vi "Acc G test.vi"() -> ()   [LabVIEW 2013]
uses:
  <vilib>/Utility/error.llb/DialogType.ctl
  <vilib>/DAQmx/read.llb/DAQmx Read (Analog 1D Wfm NChan NSamp).vi
  <vilib>/DAQmx/configure/timing.llb/DAQmx Timing (Sample Clock).vi
  <vilib>/DAQmx/configure/task.llb/DAQmx Configure Logging (TDMS).vi
  <vilib>/measure/mascope.llb/Transition Measurements N chan.vi
  <vilib>/DAQmx/create/channels.llb/DAQmx Create Channel (AI-Voltage-Basic).vi
  <vilib>/DAQmx/configure/trigger.llb/DAQmx Start Trigger (Digital Edge).vi
  <vilib>/DAQmx/configure/trigger.llb/DAQmx Start Trigger (Analog Edge).vi
  <vilib>/DAQmx/configure/trigger.llb/DAQmx Reference Trigger (Digital Edge).vi
  <vilib>/DAQmx/configure/trigger.llb/DAQmx Reference Trigger (Analog Edge).vi
  <vilib>/DAQmx/miscellaneous.llb/DAQmx Fill In Error Info.vi
  <resource>/objmgr/daqmx.rc
  <vilib>/measure/NI_MAPro.lvlib
panel:
  out "Y max":dbl caption="Y 최대" format="%0.2f"
  out "웨이브폼 그래프":waveform(dbl)[](graph)
  in  "샘플 개수":i32=100
  in  "트리거 타입":T1(tab)
  in  "에지":i32(ring)=10280 items=["상승"=10280, "하강"=10171]
  in  "디지털 트리거 소스":tag
  in  "레벨(V)":dbl format="%0.2f"
  in  "히스테리시스(V)":dbl
  in  "기울기":i32(ring)=10280 items=["상승"=10280, "하강"=10171]
  in  "아날로그 트리거 소스":string="APFI0"
  in  "디지털 참조 트리거 소스":tag
  in  "에지 2":i32(ring)=10280 items=["상승"=10280, "하강"=10171]
  in  "트리거 이전 샘플":u32
  in  "아날로그 참조 트리거 소스":string="APFI0"
  in  "기울기 2":i32(ring)=10280 items=["상승"=10280, "하강"=10171]
  in  "레벨(V) 2":dbl format="%0.2f"
  in  "트리거 이전 샘플 2":u32
  in  "TDMS 파일 경로":path
  in  "샘플 속도":dbl=1000.0
  in  "샘플 클럭 소스":tag="OnboardClock"
  in  "터미널 설정":i32(ring)=-1 items=["기본값"=-1, "RSE"=10083, "NRSE"=10078, "차동"=10106, "유사 차동"=12529]
  in  "최대 전압":dbl=5.0
  in  "최소 전압":dbl=-5.0
  in  "물리적인 채널":tag="Dev1/ai0"
  out "실제 샘플 속도":dbl=1000.0 format="%0.2f"
  in  "로깅 모드":i32(ring)=10231 items=["Off"=10231, "로그 및 읽기"=15842]
  # "시작 트리거를 설정하고 사용하려면 위의 탭이 있어야 합니다.  일부 하드웨어는 트리거를 지원하지 않습니다. 더 자세한 정보는 디바이스 문서를 참조하십시오."
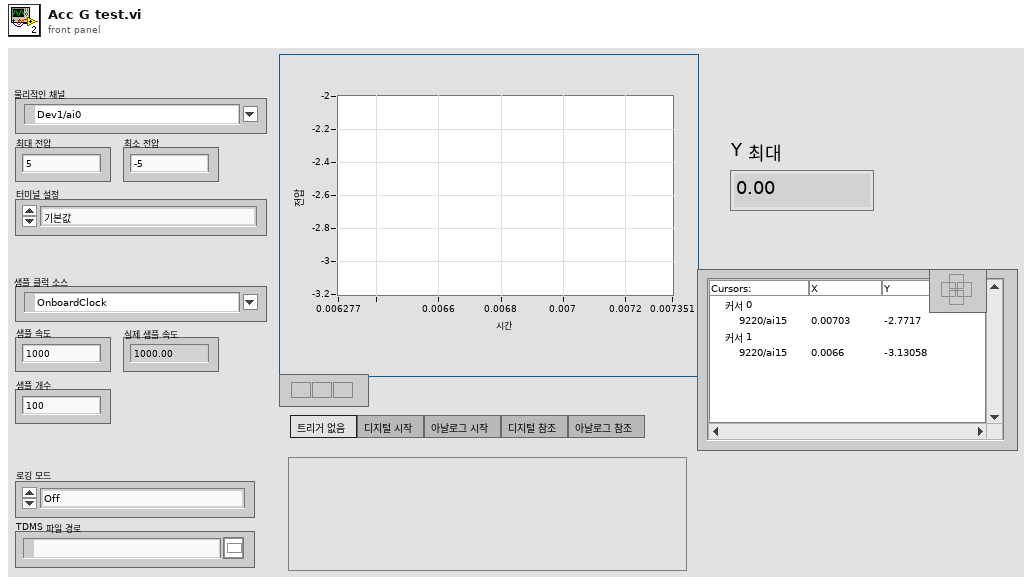
[diagram p1: front panel]
types:
  T1 = enum32{"No Trigger", "Digital Start", "Analog Start", "Digital Ref", "Analog Ref"}
  T2 = typedef "DialogType.ctl" = u16
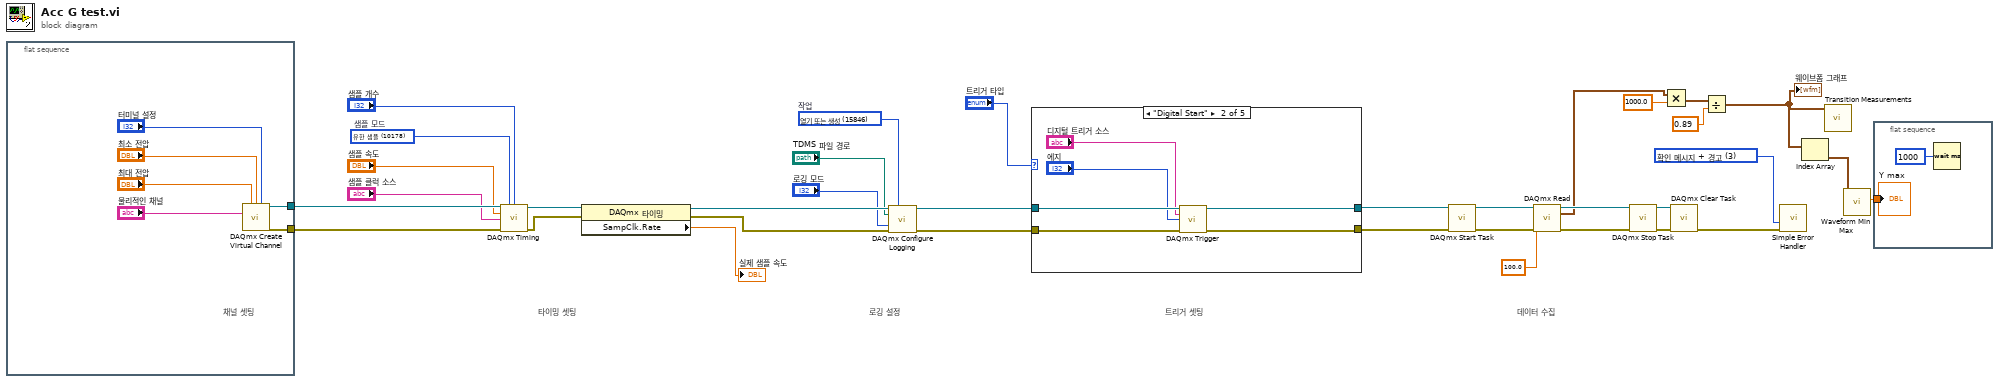
[diagram p0: block diagram]
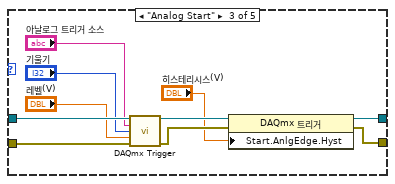
[diagram p3: hidden frame]
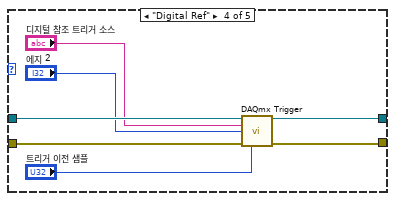
[diagram p4: hidden frame]
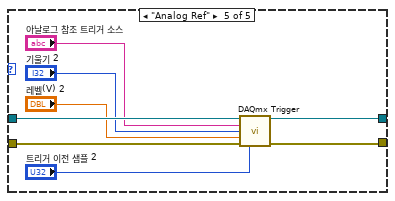
[diagram p5: hidden frame]
diagram:
  w9 = T2 3 items=["대화 상자 없음", "확인 메시지", "메시지 지속 또는 정지", "확인 메시지 + 경고", "지속/정지 + 경고"] ("대화 상자 타입 (확인 메시지:1)")
  w28 = 15846 items=["열기"=10437, "열기 또는 생성"=15846, "생성 또는 대체"=15847, "생성"=15848]  # 작업
  w33 = 10178 items=["유한 샘플"=10178, "연속 샘플"=10123, "하드웨어 타이밍에 의한 단일 포인트"=12522]  # 샘플 모드
  # "데이터 수집"
  # "트리거 셋팅"
  # "타이밍 셋팅"
  # "로깅 설정"
  n1 = flat-sequence {
    tunnel: [w41] -> w32
    tunnel: [w40] -> w31
    frame #0 {
      # "채널 셋팅"
      n2 = call-poly <vilib>:"DAQmx Create Virtual Channel.vi"("maximum value"="최대 전압", "minimum value"="최소 전압", "input terminal configuration"="터미널 설정", "physical channels"="물리적인 채널") -> ("task out"=w40:refnum<k21>, "error out"=w41:errorcluster)  [unwired: 10 in]
    }
  }
  n3 = call-poly <vilib>:"DAQmx Timing.vi"("task/channels in"=w31, "sample mode"=w33, "samples per channel"="샘플 개수", "rate"="샘플 속도", "source"="샘플 클럭 소스", "error in"=w32) -> ("task out"=w35:refnum<k21>, "error out"=w34:errorcluster)  [unwired: 8 in]
  n4 = property class="DAQmx 타이밍"(reference=w35, error in=w34) -> (reference out=w30:refnum<k21>, error out=w29:errorcluster, "SampClk.Rate"=→"실제 샘플 속도":dbl)
  n5 = call-poly <vilib>:"DAQmx Configure Logging.vi"("task/channels in"=w30, "operation"=w28, "file path"="TDMS 파일 경로", "logging mode"="로깅 모드", "error in"=w29) -> ("task out"=w27:refnum<k21>, "error out"=w26:errorcluster)  [unwired: 9 in]
  n6 = case shown="\"Digital Start\"" "트리거 타입" {
    tunnel: w27 -> [w43 w49 w59 w66 w74]
    tunnel: w26 -> [w42 w48 w58 w65 w73]
    tunnel: [w43 w47 w56 w64 w68] -> w25
    tunnel: [w42 w46 w55 w63 w69] -> w24
    frame "No Trigger", Default {
    }
    frame "Digital Start" {
      n7 = call-poly <vilib>:"DAQmx Trigger.vi"("task/channels in"=w49, "source"="디지털 트리거 소스", "edge"="에지", "error in"=w48) -> ("task out"=w47:refnum<k21>, "error out"=w46:errorcluster)  [unwired: 10 in]
    }
    frame "Analog Start" {
      n8 = call-poly <vilib>:"DAQmx Trigger.vi"("task/channels in"=w59, "source"="아날로그 트리거 소스", "slope"="기울기", "level"="레벨(V)", "error in"=w58) -> ("task out"=w54:refnum<k21>, "error out"=w53:errorcluster)  [unwired: 9 in]
      n9 = property class="DAQmx 트리거"(reference=w54, error in=w53, "Start.AnlgEdge.Hyst"="히스테리시스(V)") -> (reference out=w56:refnum<k21>, error out=w55:errorcluster)
    }
    frame "Digital Ref" {
      n10 = call-poly <vilib>:"DAQmx Trigger.vi"("task/channels in"=w66, "source"="디지털 참조 트리거 소스", "edge"="에지 2", "error in"=w65, "pretrigger samples per channel"="트리거 이전 샘플") -> ("task out"=w64:refnum<k21>, "error out"=w63:errorcluster)  [unwired: 9 in]
    }
    frame "Analog Ref" {
      n11 = call-poly <vilib>:"DAQmx Trigger.vi"("task/channels in"=w74, "source"="아날로그 참조 트리거 소스", "slope"="기울기 2", "level"="레벨(V) 2", "error in"=w73, "pretrigger samples per channel"="트리거 이전 샘플 2") -> ("task out"=w68:refnum<k21>, "error out"=w69:errorcluster)  [unwired: 8 in]
    }
  }
  n12 = call <vilib>:"DAQmx Start Task.vi"("task/channels in"=w25, "error in"=w24) -> ("task out"=w23:refnum<k21>, "error out"=w22:errorcluster)  [unwired: 12 in]
  n13 = call-poly <vilib>:"DAQmx Read.vi"("task/channels in"=w23, "timeout"=100.0, "error in"=w22) -> ("task out"=w11:refnum<k21>, "data"=w6:waveform(dbl)[], "error out"=w10:errorcluster)  [unwired: 10 in]
  n14 = call <vilib>:"DAQmx Stop Task.vi"("task/channels in"=w11, "error in"=w10) -> ("task out"=w13:refnum<k21>, "error out"=w12:errorcluster)  [unwired: 12 in]
  n15 = Multiply(x=w6, y=1000.0) -> (x*y=w5:waveform(dbl)[])
  n16 = call <vilib>:"DAQmx Clear Task.vi"("task in"=w13, "error in"=w12) -> ("error out"=w21:errorcluster)  [unwired: 13 in]
  n17 = Divide(x=w5, y=0.89) -> (x/y=w3:waveform(dbl)[])
  "웨이브폼 그래프" <- w3
  n18 = call <vilib>:"Simple Error Handler.vi"("type of dialog (OK msg:1)"=w9, "error in (no error)"=w21) -> ()  [unwired: 3 in, 5 out]
  n19 = Index Array(array=w3) -> (element=w2:waveform(dbl))  [unwired: 1 in]
  n20 = call-poly <vilib>:"Transition Measurements.vi"("signal(s) in"=w3) -> ()  [unwired: 5 in, 6 out]
  n21 = call <vilib>:"Waveform Min Max.vi"("waveform in"=w2) -> ("Y max"=w1:dbl)  [unwired: 5 in, 5 out]
  n22 = flat-sequence {
    tunnel: w1 -> [w76]
    frame #0 {
      n23 = Wait (ms)(milliseconds to wait=u32 1000 ("대기 시간(ms)")) -> ()  [unwired: 1 out]
      "Y max" <- w76
    }
  }
